vi "Do.vi"(8 "error in (no error)":errorcluster, 9 "Events":refnum<class "Events.lvclass">, 10 "Message Loop Data in":T1, 11 "IInternalRequest in":refnum<class "EventHandler JSON.lvclass">) -> (0 "error out":errorcluster, 2 "Message Loop Data out":T1, 3 "IInternalRequest out":refnum<class "EventHandler JSON.lvclass">)   [LabVIEW 2020, in "wamplv.lvlib" / "EventHandler JSON.lvclass"]
uses:
  EventHandler JSON.lvclass
  EventHandler JSON.lvclass/EventHandler JSON.ctl
  WAMP Client/Private/TypeDef/EVENT payload (JSON).ctl
  wamplv.lvlib
  Events/JsonEvents/JsonEvents.lvclass
  Utils/Utils.lvclass
  Message loop classes/Subscription details/SubscriptionDetails JSON/SubscriptionDetails JSON.lvclass
  SerialisedMessages/JSONMessage/WampMessage JSON.lvclass
  WAMP Client/Private/TypeDef/Publish Requests Map.ctl
  WAMP Client/Private/TypeDef/Endpoint Data.ctl
  Call/ICallRequest/ICallRequest.lvclass
  WAMP Client/Private/TypeDef/CALL Request Map.ctl
  WAMP Client/Private/TypeDef/SUBSCRIBE Requests Map.ctl
  WAMP Client/Private/TypeDef/Subscriptions Map.ctl
  WAMP Client/Private/TypeDef/Unsubscribe Requests Map.ctl
  WAMP Client/Private/TypeDef/Unregister requests map.ctl
  WAMP Client/Private/TypeDef/Message Loop Data.ctl
  Events/EventsParent/Events.lvclass
  Subscribe/ISubscribe/ISubscribe.lvclass
  Publish/IPublish/IPublish.lvclass
  Message loop classes/Subscription details/SubscriptionDetailsParent/SubscriptionDetailsParent.lvclass
  Unsubscribe/IUnsubscribe/IUnsubscribe.lvclass
  Register/IRegister/IRegister.lvclass
  Unregister/IUnregister/IUnregister.lvclass
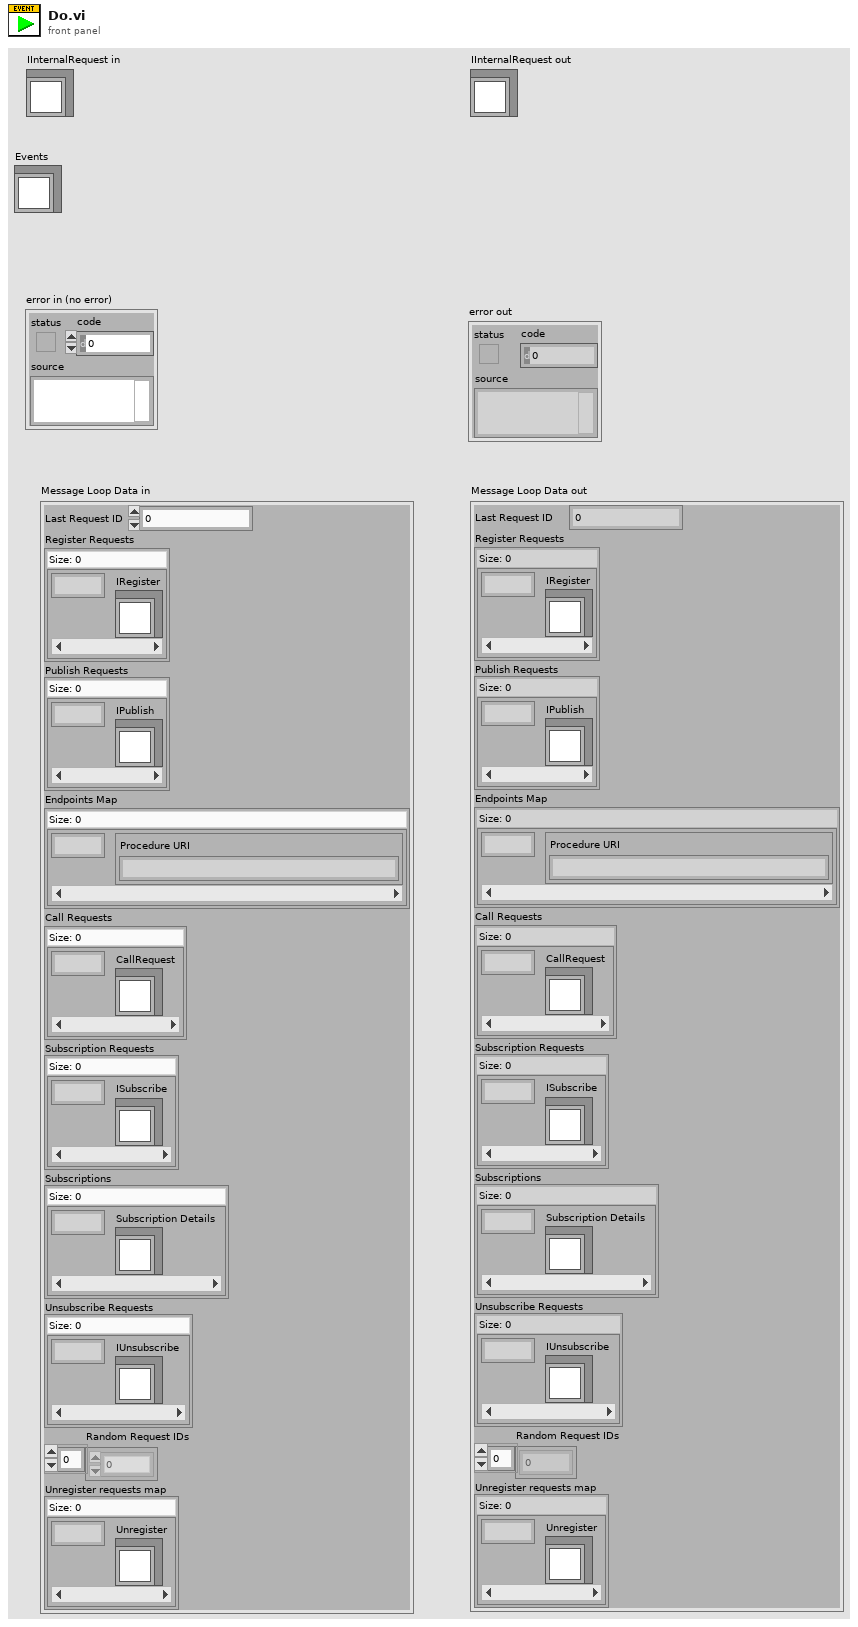
[diagram p1: front panel]
types:
  T1 = typedef "wamplv.lvlib/Message Loop Data.ctl" = cluster{"Last Request ID":u64, "Register Requests":map{u64, refnum<class "IRegister.lvclass">}, "Publish Requests":T2, "Endpoints Map":map{u64, T3}, "Call Requests":T4, "Subscription Requests":T5, "Subscriptions":T6, "Unsubscribe Requests":T7, "Random Request IDs":u64[], "Unregister requests map":T8}
  T2 = typedef "wamplv.lvlib/Publish Requests Map.ctl" = map{u64, refnum<class "IPublish.lvclass">}
  T3 = typedef "wamplv.lvlib/Endpoint Data.ctl" = cluster{"Procedure URI":string}
  T4 = typedef "wamplv.lvlib/CALL Request Map.ctl" = map{u64, refnum<class "ICallRequest.lvclass">}
  T5 = typedef "wamplv.lvlib/SUBSCRIBE Requests Map.ctl" = map{u64, refnum<class "ISubscribe.lvclass">}
  T6 = typedef "wamplv.lvlib/Subscriptions Map.ctl" = map{u64, refnum<class "SubscriptionDetailsParent.lvclass">}
  T7 = typedef "wamplv.lvlib/Unsubscribe Requests Map.ctl" = map{u64, refnum<class "IUnsubscribe.lvclass">}
  T8 = typedef "wamplv.lvlib/Unregister requests map.ctl" = map{u64, refnum<class "IUnregister.lvclass">}
  T9 = typedef "wamplv.lvlib/EVENT payload (JSON).ctl" = cluster{"Publication ID":u64, "Topic":string, "Arguments Payload":string, "ArgumentKw Payload":string, "Details":string}
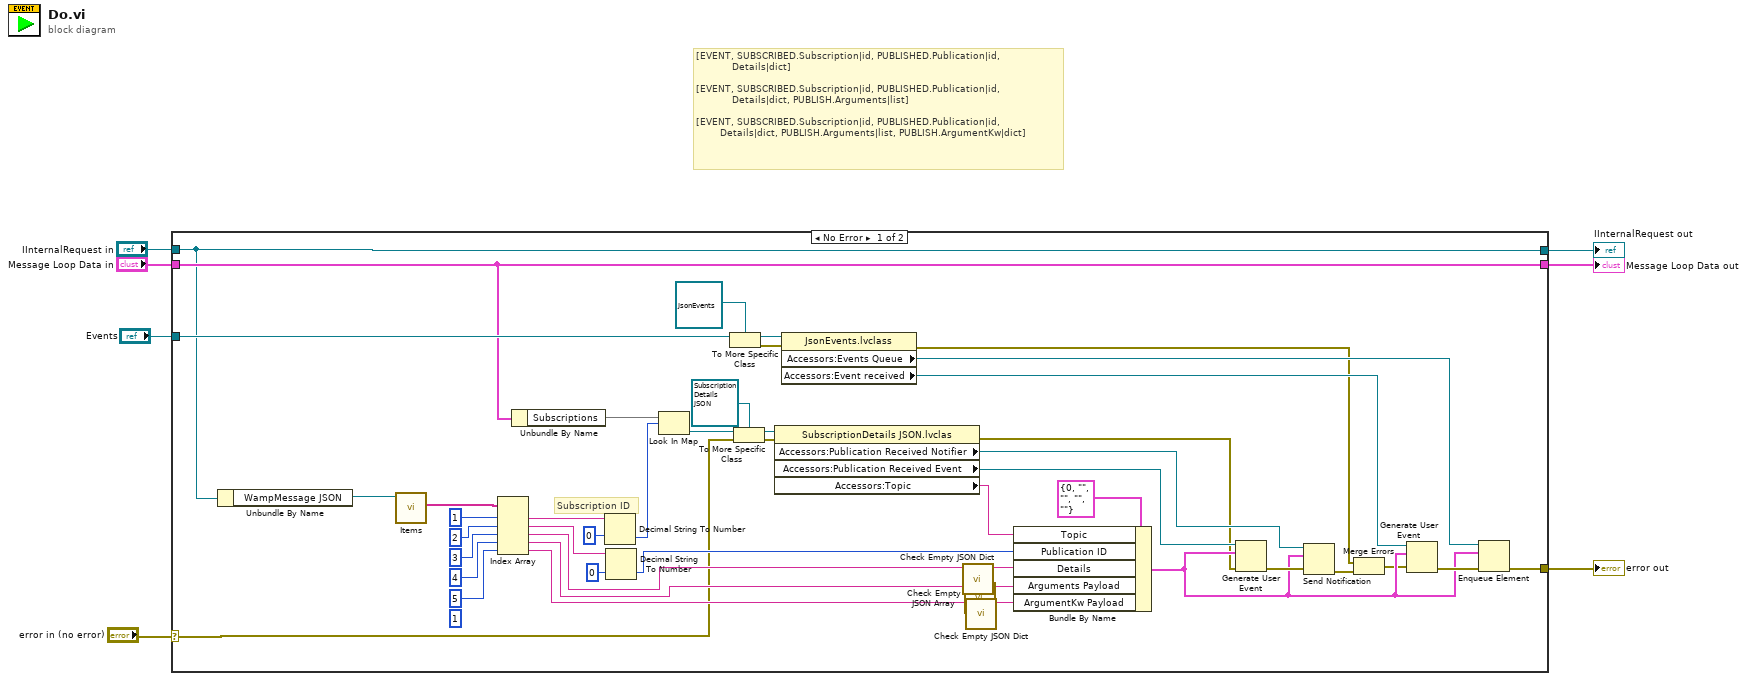
[diagram p0: block diagram]
diagram:
  # "[EVENT, SUBSCRIBED.Subscription|id, PUBLISHED.Publication|id,\n            Details|dict]\n\n[EVENT, SUBSCRIBED.Subscription|id, PUBLISHED.Publication|id,\n            Details|dict, PUBLISH.Arguments|list]\n\n[EVENT, SUBSCRIBED.Subscription|id, PUBLISHED.Publication|id,\n        Details|dict, PUBLISH.Arguments|list, PUBLISH.ArgumentKw|dict]"
  n1 = case shown="No Error" "error in (no error)" {
    selector: "error in (no error)" -> [w8 w53]
    tunnel: "Message Loop Data in" -> [w11 w54]
    tunnel: "Events" -> [w44 _]
    tunnel: "IInternalRequest in" -> [w10 w55]
    tunnel: [w10 w55] -> w3
    tunnel: [w12 w53] -> w2
    tunnel: [w11 w54] -> w1
    frame No Error {
      (unwired) 1 ("index")
      # "Subscription ID"
      n2 = Unbundle By Name(w10) -> ("WampMessage JSON"=w9:refnum<class "WampMessage JSON.lvclass">)
      n3 = call-dynamic "Items.vi"("JSONMessage in"=w9) -> ("<JSON>Elements"=w37:string[])  [unwired: 9 in, 1 out]
      n4 = Index Array(array=w37, index #1=1 ("index"), index #2=2 ("index"), index #3=3 ("index"), index #4=4 ("index"), index #5=5 ("index")) -> (element #1=w52:string, element #2=w29:string, element #3=w27:string, element #4=w26:string, element #5=w23:string)
      n5 = Unbundle By Name(w11) -> ("Subscriptions"=w46:T6)
      n6 = Decimal String To Number(string=w52, default (0L)=u64 0) -> (number=w49:u64)  [unwired: 1 in, 1 out]
      n7 = Decimal String To Number(string=w29, default (0L)=u64 0) -> (number=w34:u64)  [unwired: 1 in, 1 out]
      n8 = Look In Map(map=w46, key=w49) -> (value=w22:refnum<class "SubscriptionDetailsParent.lvclass">)  [unwired: 1 in, 1 out]
      n9 = To More Specific Class(target class=refnum<class "JsonEvents.lvclass"> refnum ("wamplv.lvlib:JsonEvents.lvclass"), reference=w44) -> (specific class reference=w43:refnum<class "JsonEvents.lvclass">, error out=w39:errorcluster)  [unwired: 1 in]
      n10 = To More Specific Class(target class=refnum<class "SubscriptionDetails JSON.lvclass"> refnum ("wamplv.lvlib:SubscriptionDetails JSON.lvclass"), reference=w22, error in=w8) -> (specific class reference=w20:refnum<class "SubscriptionDetails JSON.lvclass">, error out=w16:errorcluster)
      n11 = property class="SubscriptionDetails JSON.lvclas"(reference=w20, error in=w16) -> (error out=w15:errorcluster, "Accessors:Publication Received Notifier"=w17:refnum<notifier>, "Accessors:Publication Received Event"=w18:refnum<user-event>, "Accessors:Topic"=w19:string)  [unwired: 1 out]
      n12 = property class="JsonEvents.lvclass"(reference=w43, error in=w39) -> (error out=w38:errorcluster, "Accessors:Events Queue"=w41:refnum<queue>, "Accessors:Event received "=w40:refnum<user-event>)  [unwired: 1 out]
      n13 = call "Check Empty JSON Dict.vi"("JSON in"=w27) -> ("JSON out"=w28:string)  [unwired: 10 in]
      n14 = call "Check Empty JSON Array.vi"("JSON in"=w26) -> ("JSON out"=w25:string)  [unwired: 10 in]
      n15 = call "Check Empty JSON Dict.vi"("JSON in"=w23) -> ("JSON out"=w24:string)  [unwired: 10 in]
      n16 = Bundle By Name(cluster=T9 {"Publication ID"=0, "Topic"="", "Arguments Payload"="", "ArgumentKw Payload"="", "Details"=""} ("Cluster"), "Topic"=w19, "Publication ID"=w34, "Details"=w28, "Arguments Payload"=w25, "ArgumentKw Payload"=w24) -> (w36:T9)
      n17 = Generate User Event(user event=w18, event data cluster=w36, error in=w15) -> (error out=w45:errorcluster)  [unwired: 1 in, 1 out]
      n18 = Send Notification(notification=w36, notifier=w17, error in (no error)=w45) -> (error out=w14:errorcluster)  [unwired: 1 out]
      n19 = Merge Errors(w38, w14) -> (w13:errorcluster)
      n20 = Generate User Event(user event=w40, event data cluster=w36, error in=w13) -> (error out=w47:errorcluster)  [unwired: 1 in, 1 out]
      n21 = Enqueue Element(queue=w41, element=w36, error in (no error)=w47) -> (error out=w12:errorcluster)  [unwired: 1 in, 2 out]
    }
    frame Error {
    }
  }
  "error out" <- w2
  "IInternalRequest out" <- w3
  "Message Loop Data out" <- w1
